vi "Send_Email_Attach.vi"(6 "Attachment Path":path=path "C:/Users/Simon/Dropbox/Medimatic/Project Ver. LV2011/Journaler/DBT 010360-2190 11-04-2012.xls", 7 "Recipient's Name":string, 8 "Error In":errorcluster, 9 "Body":string="Journal", 10 "Subject":string="Journal from DM2000 Digital", 11 "Recipient's Email Address":string="kamronn@gmail.com") -> (0 "Error Out":errorcluster)   [LabVIEW 2013, in "main.lvlib"]
uses:
  main.lvlib
  <vilib>/regexp/Match Regular Expression.xnode
panel:
  in  "Sender's Name":string="Medimatic"
  in  "Sender's Email Address":string="journal@medimatic.dk"
  in  "Enable SSL":bool
  in  "Port":i32=587
  in  "SMTP Outgoing Mail Server":string="mail.medimatic.dk"
  in  "Email Account Password":string="KodeOrd123"
  in  "Email Account ID":string="journal@medimatic.dk"
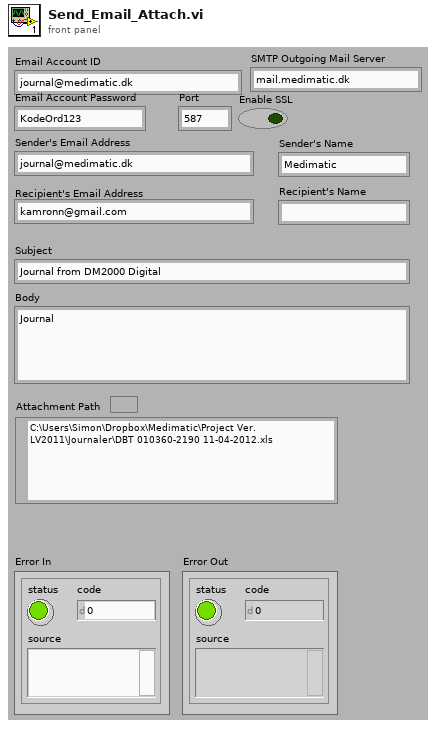
[diagram p1: front panel]
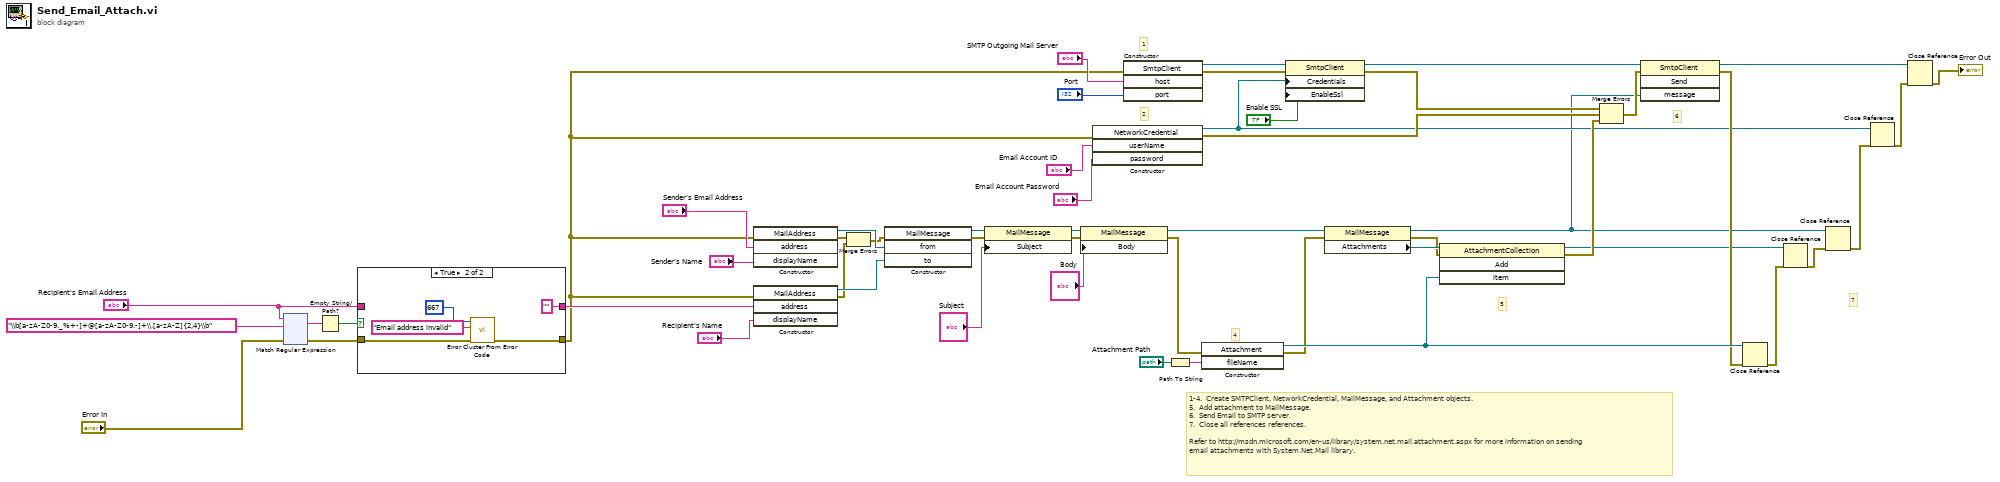
[diagram p0: block diagram]
diagram:
  # "1-4.  Create SMTPClient, NetworkCredential, MailMessage, and Attachment objects.\n5.  Add attachment to MailMessage.\n6.  Send Email to SMTP server.\n7.  Close all references references.\n\nRefer to http://msdn.microsoft.com/en-us/library/system.net.mail.attachment.aspx for more information on sending\nemail attachments with System.Net.Mail library."
  # "7"
  # "6"
  # "5"
  # "4"
  # "2"
  # "1"
  n1 = xnode "Match Regular Expression"("input string"="Recipient's Email Address", "regular expression"="\\b[a-zA-Z0-9._%+-]+@[a-zA-Z0-9.-]+\\.[a-zA-Z]{2,4}\\b", "error in"="Error In") -> ("whole match"=w4:string, "error out"=w5:errorcluster)  [unwired: 3 in, 3 out]
  n2 = Empty String/Path?(string/path=w4) -> (empty?=w6:bool)
  n3 = case shown="True" w6 {
    tunnel: w5 -> [w54 w59]
    tunnel: [w54 w56] -> w1
    tunnel: "Recipient's Email Address" -> [w53 _]
    tunnel: [w53 "" ("Recipient's Email Address")] -> w3
    frame False {
    }
    frame True {
      n4 = call <vilib>:"Error Cluster From Error Code.vi"("error in (no error)"=w59, "error message (\"\")"="Email address invalid" ("error message (\"\")"), "error code (0)"=667) -> ("error out"=w56:errorcluster)  [unwired: 6 in]
    }
  }
  n5 = constructor class="MailAddress"(error in=w1, "address"="Sender's Email Address", "displayName"="Sender's Name") -> (reference out=w14:refnum<k24>, error out=w11:errorcluster)  [unwired: 2 in, 3 out]
  n6 = constructor class="MailAddress"(error in=w1, "address"=w3, "displayName"="Recipient's Name") -> (reference out=w26:refnum<k24>, error out=w9:errorcluster)  [unwired: 2 in, 3 out]
  n7 = Merge Errors(w11, w9) -> (w10:errorcluster)
  n8 = constructor class="MailMessage"(error in=w10, "from"=w14, "to"=w26) -> (reference out=w18:refnum<k24>, error out=w13:errorcluster)  [unwired: 2 in, 3 out]
  n9 = property class="MailMessage"(reference=w18, error in=w13, "Subject"="Subject") -> (reference out=w19:refnum<k24>, error out=w25:errorcluster)
  n10 = property class="MailMessage"(reference=w19, error in=w25, "Body"="Body") -> (reference out=w16:refnum<k24>, error out=w15:errorcluster)
  n11 = constructor class="NetworkCredential"(error in=w1, "userName"="Email Account ID", "password"="Email Account Password") -> (reference out=w29:refnum<k24>, error out=w37:errorcluster)  [unwired: 2 in, 3 out]
  n12 = constructor class="SmtpClient"(error in=w1, "host"="SMTP Outgoing Mail Server", "port"="Port") -> (reference out=w52:refnum<k24>, error out=w41:errorcluster)  [unwired: 2 in, 3 out]
  n13 = Path To String(path="Attachment Path") -> (string=w44:string)
  n14 = constructor class="Attachment"(error in=w15, "fileName"=w44) -> (reference out=w35:refnum<k24>, error out=w17:errorcluster)  [unwired: 2 in, 2 out]
  n15 = property class="SmtpClient"(reference=w52, error in=w41, "Credentials"=w29, "EnableSsl"="Enable SSL") -> (reference out=w51:refnum<k24>, error out=w40:errorcluster)
  n16 = property class="MailMessage"(reference=w16, error in=w17) -> (reference out=w27:refnum<k24>, error out=w42:errorcluster, "Attachments"=w43:refnum<k24>)
  n17 = invoke class="AttachmentCollection" method="Add"(reference=w43, error in=w42, "item"=w35) -> (reference out=w33:refnum<k24>, error out=w36:errorcluster)  [unwired: 1 in, 2 out]
  n18 = Merge Errors(w40, w37, w36) -> (w39:errorcluster)
  n19 = invoke class="SmtpClient" method="Send"(reference=w51, error in=w39, "message"=w27) -> (reference out=w38:refnum<k24>, error out=w34:errorcluster)  [unwired: 1 in, 2 out]
  n20 = Close Reference(reference=w35, error in (no error)=w34) -> (error out=w32:errorcluster)
  n21 = Close Reference(reference=w33, error in (no error)=w32) -> (error out=w31:errorcluster)
  n22 = Close Reference(reference=w27, error in (no error)=w31) -> (error out=w30:errorcluster)
  n23 = Close Reference(reference=w29, error in (no error)=w30) -> (error out=w28:errorcluster)
  n24 = Close Reference(reference=w38, error in (no error)=w28) -> (error out=→"Error Out":errorcluster)
